vi "brake.vi"(5 "Motors 2":i32=-1, 7 "Motors":i32=-1, 10 "NXT/EV3":T1) -> (2 "NXT/EV3 2":T1)   [LabVIEW 2016]
uses:
  <vilib>/NXT/Subs/LVHSConnector.ctl
  <vilib>/NXT/LegoClasses/BrickReference/BrickReference.lvclass
  <vilib>/NXT/NXTIO Xnodes/NXTIONodeSubVIs/NXTStopMotors.vi
  <vilib>/NXT/NXTIO Xnodes/NXTIOXNode/NXTIO.xnode
  <vilib>/NXT/Block Support/NXT_OutputPort.ctl
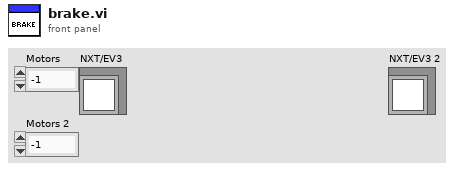
[diagram p1: front panel]
types:
  T1 = typedef "LVHSConnector.ctl" = refnum<class "BrickReference.lvclass">
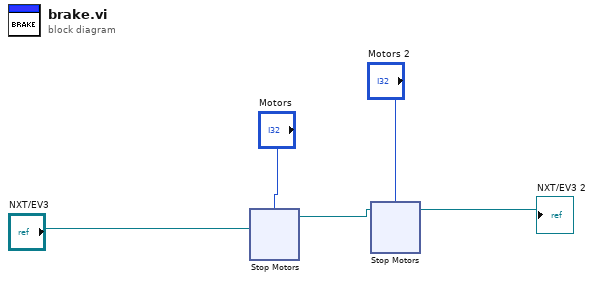
[diagram p0: block diagram]
diagram:
  n1 = xnode "Stop Motors"("Motors"="Motors", "NXT/EV3"="NXT/EV3") -> ("NXT/EV3"=w3:T1)
  n2 = xnode "Stop Motors"("Motors"="Motors 2", "NXT/EV3"=w3) -> ("NXT/EV3"=→"NXT/EV3 2":T1)
